vi "ReadWriteServiceRequest.vi"(4 "Service ROS":T2={"topic port"=1236, "Node"="/labview", "topic"="/robot/head/command_head_nod", "type"="std_msgs/Bool", "node port"=7000, "error "={"status"=FALSE, "code"=0, "source"=""}, "Direction"=enum."Publisher", "APIs"=[], "Update (ms)"=1, "write queue"=1}, 5 "Error in":string, 6 "data":string, 7 "Log in":T4[](array[typedef])) -> (0 "Error out":string, 1 "String Read":string, 2 "Log":T4[](array[typedef]), 3 "MyState":T5)   [LabVIEW 2010]
uses:
  MyState.ctl
  ROSLog.ctl
  SubVIs/_ROSDirection.ctl
  SubVIs/_ROSControl.ctl
panel:
  out "Array":errorcluster[](array[cluster])
  out "Connections":T1(array[cluster])
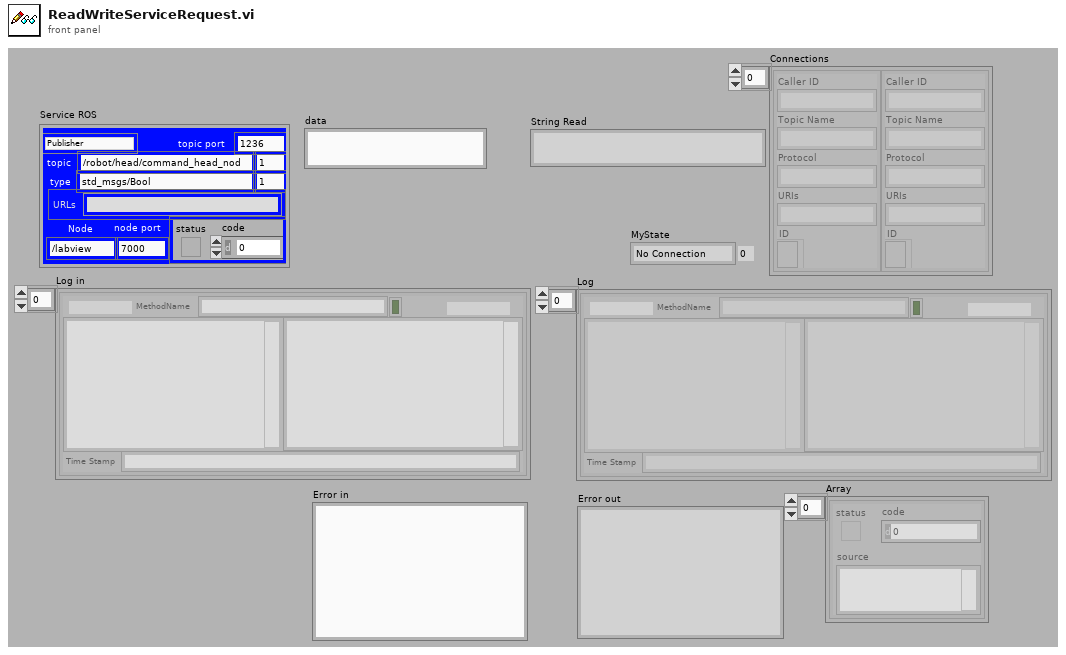
[diagram p1: front panel]
types:
  T1 = cluster{"Caller ID":string, "Topic Name":string, "Protocol":string, "URIs":string, "ID":refnum<k5>}[]
  T2 = typedef "_ROSControl.ctl" = cluster{"topic port":u16, "Node":string, "topic":string, "type":string, "node port":u32, "error ":errorcluster, "Direction":T3, "APIs":string[], "Update (ms)":u16, "write queue":u16}
  T3 = typedef "_ROSDirection.ctl" = enum16{"Node", "Publisher", "Subscriber", "Service Client"}
  T4 = typedef "ROSLog.ctl" = cluster{"Sent":string, "Reply":string, "MethodName":string, "success":bool, "Dir1":string, "Dir2":string, "Time Stamp":string}
  T5 = typedef "MyState.ctl" = enum16{"No Connection", "Registered", "Connected", "Close"}
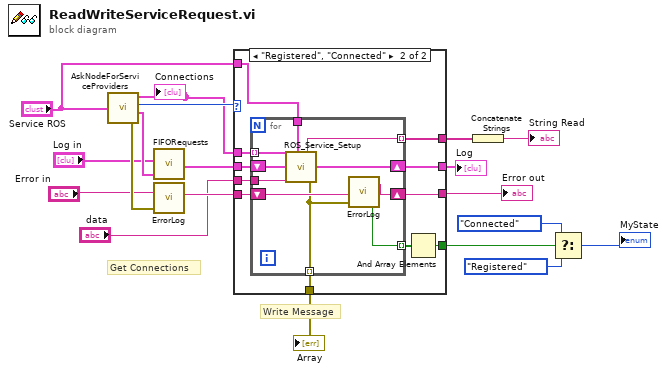
[diagram p0: block diagram]
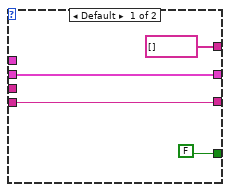
[diagram p2: hidden frame]
diagram:
  # "Write Message"
  # "Get Connections"
  n1 = call "AskNodeForServiceProviders.vi"("Service ROS"="Service ROS") -> ("Connections"=w4:T1, "MyState"=w11:T5, "Log"=w12:T4, "error out"=w14:errorcluster)
  "Connections" <- w4
  n2 = call "FIFORequests.vi"("Log"=w12, "Requests in"="Log in") -> ("Requests out"=w13:T4[])  [unwired: 1 in]
  n3 = call "ErrorLog.vi"("error in"=w14, "Error String"="Error in") -> ("String out"=w15:string)  [unwired: 1 in, 1 out]
  n4 = case shown="\"Registered\", \"Connected\"" w11 {
    tunnel: [w23 w29] -> w5
    tunnel: "data" -> [_ w34]
    tunnel: [w22 w32] -> w6
    tunnel: w4 -> [_ w31]
    tunnel: w15 -> [w23 w30]
    tunnel: w13 -> [w22 w33]
    tunnel: [string[] [] w28] -> w10
    tunnel: [FALSE ("status") w26] -> w3
    tunnel: [_ w25] -> w2
    tunnel: "Service ROS" -> [_ w24]
    frame Default {
    }
    frame "Registered", "Connected" {
      n5 = for {
        tunnel: w34 -> [w44]
        shift-right: [w42] -> w32
        shift-left: w33 -> [w43]
        tunnel: w24 -> [w41]
        tunnel: w31 -> [w40] mode=indexing
        shift-right: [w38] -> w29
        shift-left: w30 -> [w39]
        tunnel: [w37] -> w28 mode=indexing
        tunnel: [w36] -> w27 mode=indexing
        tunnel: [w35] -> w25 mode=indexing
        n6 = call "ROS_Service_Setup.vi"("Log in"=w43, "ROS"=w41, "Msg to Send"=w44, "Subscriber"=w40) -> ("Log out"=w42:T4[], "Reply"=w37:string, "error out"=w35:errorcluster)  [unwired: 1 in]
        n7 = call "ErrorLog.vi"("error in"=w35, "Error String"=w39) -> ("Success?"=w36:bool, "String out"=w38:string)  [unwired: 1 in]
      }
      n8 = And Array Elements(Boolean array=w27) -> (logical AND=w26:bool)
    }
  }
  "Error out" <- w5
  "Log" <- w6
  "Array" <- w2
  n9 = Concatenate Strings(w10) -> (→"String Read":string)
  n10 = Select(t=MyState."Connected" ("MyState"), s=w3, f=MyState."Registered" ("MyState")) -> (s? t:f=→"MyState":T5)
